vi "AES Decrypt (ECB).vi"(7 "Padding":i32(ring)=3 items=["None"=1, "PKCS7"=2, "Zeros"=3, "ANSIX923"=4, "ISO10126"=5], 8 "error in (no error)":errorcluster, 10 "Key":u8[](array[numeric]), 11 "Encrypted data in":u8[](array[numeric])) -> (0 "error out":errorcluster, 3 "Raw data out":u8[](array[numeric]))   [LabVIEW 2021, in "dotNET Crypto Symmetric Encryption.lvlib"]
doc: "Decrypt data using AES using the ECB cipher mode.\n\nThe padding mode must match the padding used to encrypt the data.\n\nNote - ECB is considered insecure as each identifcal block of data is encrypted into an identical ciphertext block."
uses:
  dotNET Crypto Symmetric Encryption.lvlib
  System.Core
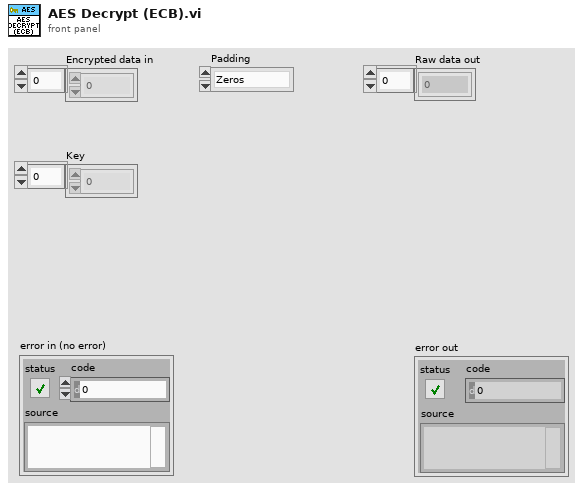
[diagram p1: front panel]
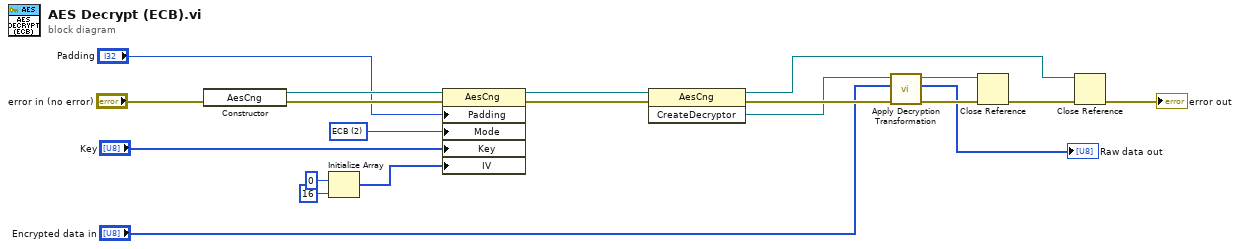
[diagram p0: block diagram]
diagram:
  w19 = 2 items=["CBC"=1, "ECB"=2, "OFB"=3, "CFB"=4, "CTS"=5] ("Mode")
  n1 = constructor class="AesCng"(error in="error in (no error)") -> (reference out=w15:refnum<k24>, error out=w16:errorcluster)  [unwired: 2 in, 1 out]
  n2 = Initialize Array(u8 0, 16 ("dimension size")) -> (w10:u8[])
  n3 = property class="AesCng"(reference=w15, error in=w16, "Padding"="Padding", "Mode"=w19, "Key"="Key", "IV"=w10) -> (reference out=w17:refnum<k24>, error out=w18:errorcluster)
  n4 = invoke class="AesCng" method="CreateDecryptor"(reference=w17, error in=w18) -> (reference out=w12:refnum<k24>, error out=w7:errorcluster, "CreateDecryptor"=w4:refnum<k24>)  [unwired: 1 in]
  n5 = call "Apply Decryption Transformation.vi"("error in (no error)"=w7, "Encrypted data in"="Encrypted data in", "Crypto transform in"=w4) -> ("error out"=w6:errorcluster, "Plaintext"=→"Raw data out":u8[], "Crypto transform out"=w5:refnum<k24>)  [unwired: 6 in]
  n6 = Close Reference(reference=w5, error in (no error)=w6) -> (error out=w11:errorcluster)
  n7 = Close Reference(reference=w12, error in (no error)=w11) -> (error out=→"error out":errorcluster)
